vi "DSF.Shared.Configuration.Transfer.Set Engine Offset.vi"(10 "engine offset":u64, 11 "Transfer Configuration in":refnum<class "DSF.Shared.Configuration.Transfer.lvclass">) -> (3 "Transfer Configuration out":refnum<class "DSF.Shared.Configuration.Transfer.lvclass">)   [LabVIEW 2017, in "DSF.Shared.lvlib" / "DSF.Shared.Configuration.Transfer.lvclass"]
uses:
  DSF.Shared.Configuration.Transfer.lvclass
  DSF.Shared.Configuration.Transfer.lvclass/DSF.Shared.Configuration.Transfer.ctl
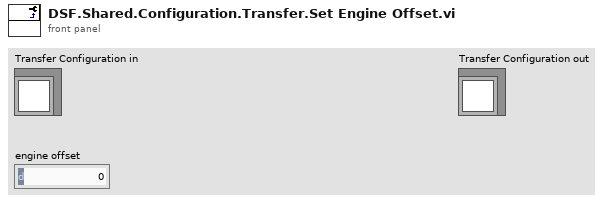
[diagram p1: front panel]
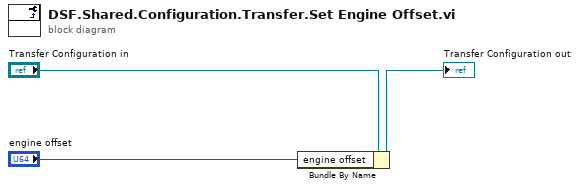
[diagram p0: block diagram]
diagram:
  n1 = Bundle By Name(cluster="Transfer Configuration in", "engine offset"="engine offset") -> (→"Transfer Configuration out":refnum<class "DSF.Shared.Configuration.Transfer.lvclass">)
